vi "axisValue.vi"() -> ()   [LabVIEW 2016]
panel:
  out "axis":dbl
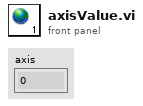
[diagram p1: front panel]
diagram:
